vi "DataFitting.vi"() -> ()   [LabVIEW 2014]
uses:
  <vilib>/gmath/SpecialFunctions.llb/Factorial.vi
  <vilib>/imath/engines/lvmath2/RunTimeEngine/Managers/WorkSpace/UID Generator.vi
  <vilib>/imath/engines/lvmath2/RunTimeEngine/BuiltInFunctions/mean/NIMS_RS=mean(RV,I32).vi
  <vilib>/imath/engines/lvmath2/RunTimeEngine/RunTimeType/NIMS_RunTimeType_From StrictType (excl LVString).vi
  <instcachedir>/0/NIMS_RunTimeType_From StrictType (excl LVString)_15A5391EEA9C4AACB9955AC755B83D29.lvgen/NIMS_RunTimeType_From StrictType (excl LVString)_15A5391EEA9C4AACB9955AC755B83D29_000.vi
  <vilib>/imath/engines/lvmath2/RunTimeEngine/LocalVariableDefStatement/MC_LocalVariableDefStatement_Display.vi
  <vilib>/imath/engines/lvmath2/RunTimeEngine/Managers/SymbolTable/Clear UID.vi
  <vilib>/imath/engines/lvmath2/RunTimeEngine/NodeEndStatement/NIMS_NodeEndStatement_Output.vi
  <instcachedir>/0/NIMS_NodeEndStatement_Output_53EC0D466D134D7ABD903AC30B43404B.lvgen/NIMS_NodeEndStatement_Output_53EC0D466D134D7ABD903AC30B43404B_004.vi
  <instcachedir>/0/NIMS_NodeEndStatement_Output_53EC0D466D134D7ABD903AC30B43404B.lvgen/NIMS_NodeEndStatement_Output_53EC0D466D134D7ABD903AC30B43404B_005.vi
  <vilib>/imath/engines/lvmath2/RunTimeEngine/ErrorHandling/NIMS_Finalize Error.vi
  <vilib>/gmath/NI_Gmath.lvlib
  <vilib>/imath/engines/lvmath2/RunTimeEngine/Managers/SymbolTable/NIMS_WorkSpace.lvlib
panel:
  out "XY Graph 2":cluster{"Array":dbl[], "y_values":dbl[]}[](graph)
  out "XY Graph":cluster{"Array":dbl[], "y_values":dbl[]}[](graph)
  in  "file path (use dialog) 2":path
  in  "file path (use dialog)":path
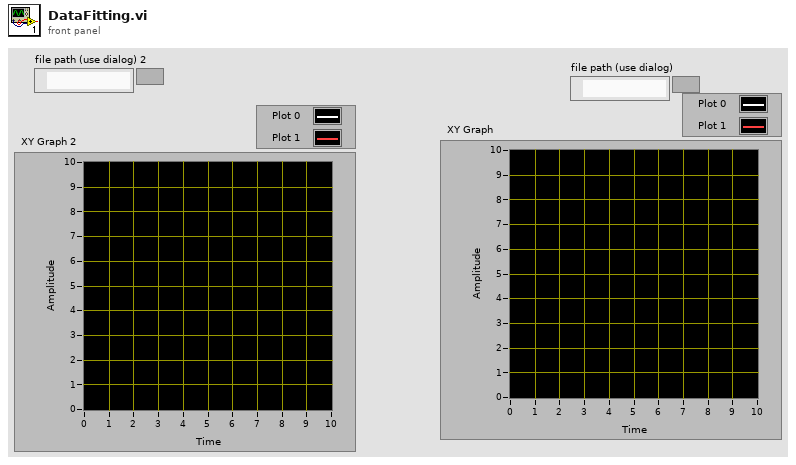
[diagram p1: front panel]
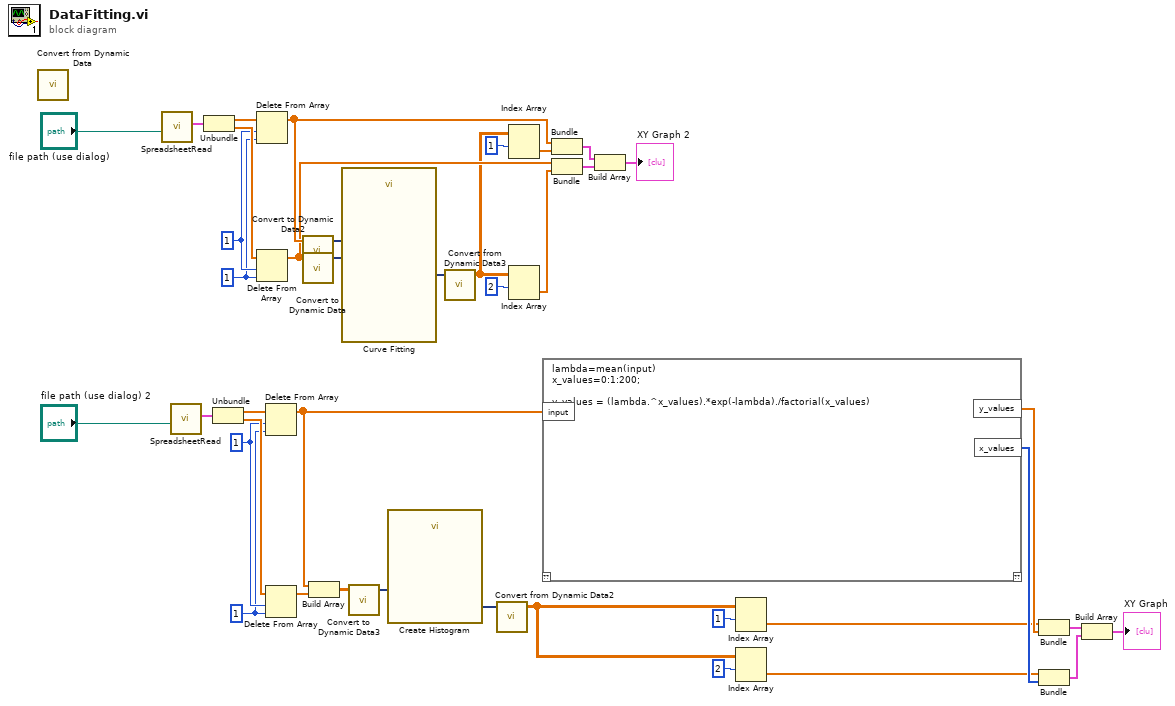
[diagram p0: block diagram]
diagram:
  w27 = 1 ("index")
  w28 = 1 ("length")
  w31 = 1 ("index")
  w32 = 1 ("length")
  n1 = call "Convert from Dynamic Data"() -> ()  [unwired: 4 in, 1 out]
  n2 = call "SpreadsheetRead.vi"("file path (use dialog)"="file path (use dialog)") -> ("output cluster"=w39:cluster{dbl[], dbl[]})  [unwired: 10 in]
  n3 = call "SpreadsheetRead.vi"("file path (use dialog)"="file path (use dialog) 2") -> ("output cluster"=w35:cluster{dbl[], dbl[]})  [unwired: 10 in]
  n4 = Unbundle(w39) -> (w34:dbl[], w33:dbl[])
  n5 = Unbundle(w35) -> (w30:dbl[], w29:dbl[])
  n6 = Delete From Array(array=w34, length=w32, index=w31) -> (array with subset deleted=w7:dbl[])  [unwired: 1 out]
  n7 = Delete From Array(array=w33, length=w32, index=w31) -> (array with subset deleted=w6:dbl[])  [unwired: 1 out]
  n8 = Delete From Array(array=w30, length=w28, index=w27) -> (array with subset deleted=w20:dbl[])  [unwired: 1 out]
  n9 = Delete From Array(array=w29, length=w28, index=w27) -> (array with subset deleted=w19:dbl[])  [unwired: 1 out]
  n10 = call "Convert to Dynamic Data2"("Array"=w7) -> ("Dynamic Data Type"=w37:dynamicdata)  [unwired: 3 in]
  n11 = call "Convert to Dynamic Data"("Array"=w6) -> ("Dynamic Data Type"=w38:dynamicdata)  [unwired: 3 in]
  n12 = Build Array(w20, w19) -> (w18:dbl[][])
  n13 = call "Curve Fitting"("Locations"=w38, "Signals"=w37) -> ("best fit"=w8:dynamicdata)  [unwired: 5 in, 4 out]
  n14 = call "Convert to Dynamic Data3"("2D Array"=w18) -> ("Dynamic Data Type"=w21:dynamicdata)  [unwired: 3 in]
  n15 = call "Create Histogram"("Signal"=w21) -> ("Histogram"=w17:dynamicdata)  [unwired: 9 in, 1 out]
  n16 = call "Convert from Dynamic Data3"("Dynamic Data Type"=w8) -> ("Array"=w3:dbl[][])  [unwired: 3 in]
  n17 = call "Convert from Dynamic Data2"("Dynamic Data Type"=w17) -> ("Array"=w15:dbl[][])  [unwired: 3 in]
  n18 = Index Array(array=w3, index (row)=1) -> (element=w1:dbl[])  [unwired: 1 in]
  n19 = Index Array(array=w3, index (row)=2) -> (element=w2:dbl[])  [unwired: 1 in]
  n20 = mathscript code="lambda=mean(input)\nx_values=0:1:200;\n\ny_values = (lambda.^x_values).*exp(-lambda)./factorial(x_values)"("input"=w20) -> ("y_values"=w24:dbl[], "x_values"=w25:i32[])  [unwired: 1 in, 1 out]
  n21 = Bundle(w7, "Array"=w1) -> (w10:cluster{dbl[], "Array":dbl[]})  [unwired: 1 in]
  n22 = Bundle(w6, "Array"=w2) -> (w9:cluster{dbl[], "Array":dbl[]})  [unwired: 1 in]
  n23 = Build Array(w10, w9) -> (→"XY Graph 2":cluster{dbl[], "Array":dbl[]}[])
  n24 = Index Array(array=w15, index (row)=1) -> (element=w16:dbl[])  [unwired: 1 in]
  n25 = Index Array(array=w15, index (row)=2) -> (element=w14:dbl[])  [unwired: 1 in]
  n26 = Bundle("Array"=w16, "y_values"=w24) -> (w23:cluster{"Array":dbl[], "y_values":dbl[]})  [unwired: 1 in]
  n27 = Bundle("Array"=w14, "x_values"=w25) -> (w22:cluster{"Array":dbl[], "x_values":i32[]})  [unwired: 1 in]
  n28 = Build Array(w23, w22) -> (→"XY Graph":cluster{"Array":dbl[], "y_values":dbl[]}[])
